vi "Manual_control.vi"() -> ()   [LabVIEW 2015]
uses:
  <vilib>/Instr/_visa.llb/VISA Configure Serial Port (Instr).vi
panel:
  out "Connected to arduino":bool
  out "Heater on":bool
  out "error out":errorcluster
  in  "Tab Control":T1(tab)
  in  "Motor distance (0-999)":string
  in  "Motor speed (NA ATM)":string
  in  "Motor acceleration (00 for constant speed) (NA ATM)":string
  in  "Step type":u16(ring) items=["Sixteenth step", "Eighth step", "Quater step", "Half step", "Full step"]
  in  "Direction":string(combo)
  in  "Motor Trigger":bool
  in  "Apply temp change":bool
  in  "Heater Temperature":string
  in  "Read temp":bool
  out "Recorded temp":string
  in  "Apply changes":bool
  in  "Amplitude set %":dbl(slide) scale=0.0..100.0
  in  "Temprature limit on":bool
  in  "Lower temp limit /°C":dbl
  in  "Upper temp limit /°C":dbl
  in  "Time limit on":bool
  in  "Time limit /s":dbl
  in  "Pluse set %":dbl(slide) scale=0.0..100.0
  in  "Manually turn spray on/off":bool
  in  "Turn off heater":bool
  in  "Stop labview functions.\n To properly disconnect \nfrom arduino use this":bool
  in  "VISA resource name":refnum<visa-resource-name>
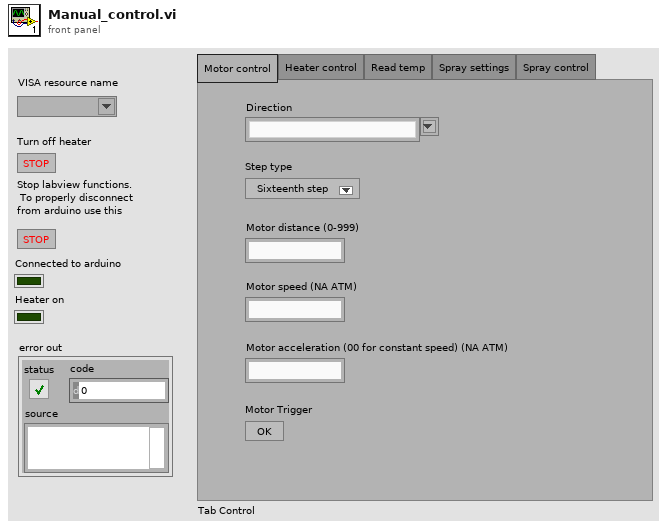
[diagram p1: front panel]
types:
  T1 = enum32{"Motor control", "Heater control", "Read temp", "Spray settings", "Spray control"}
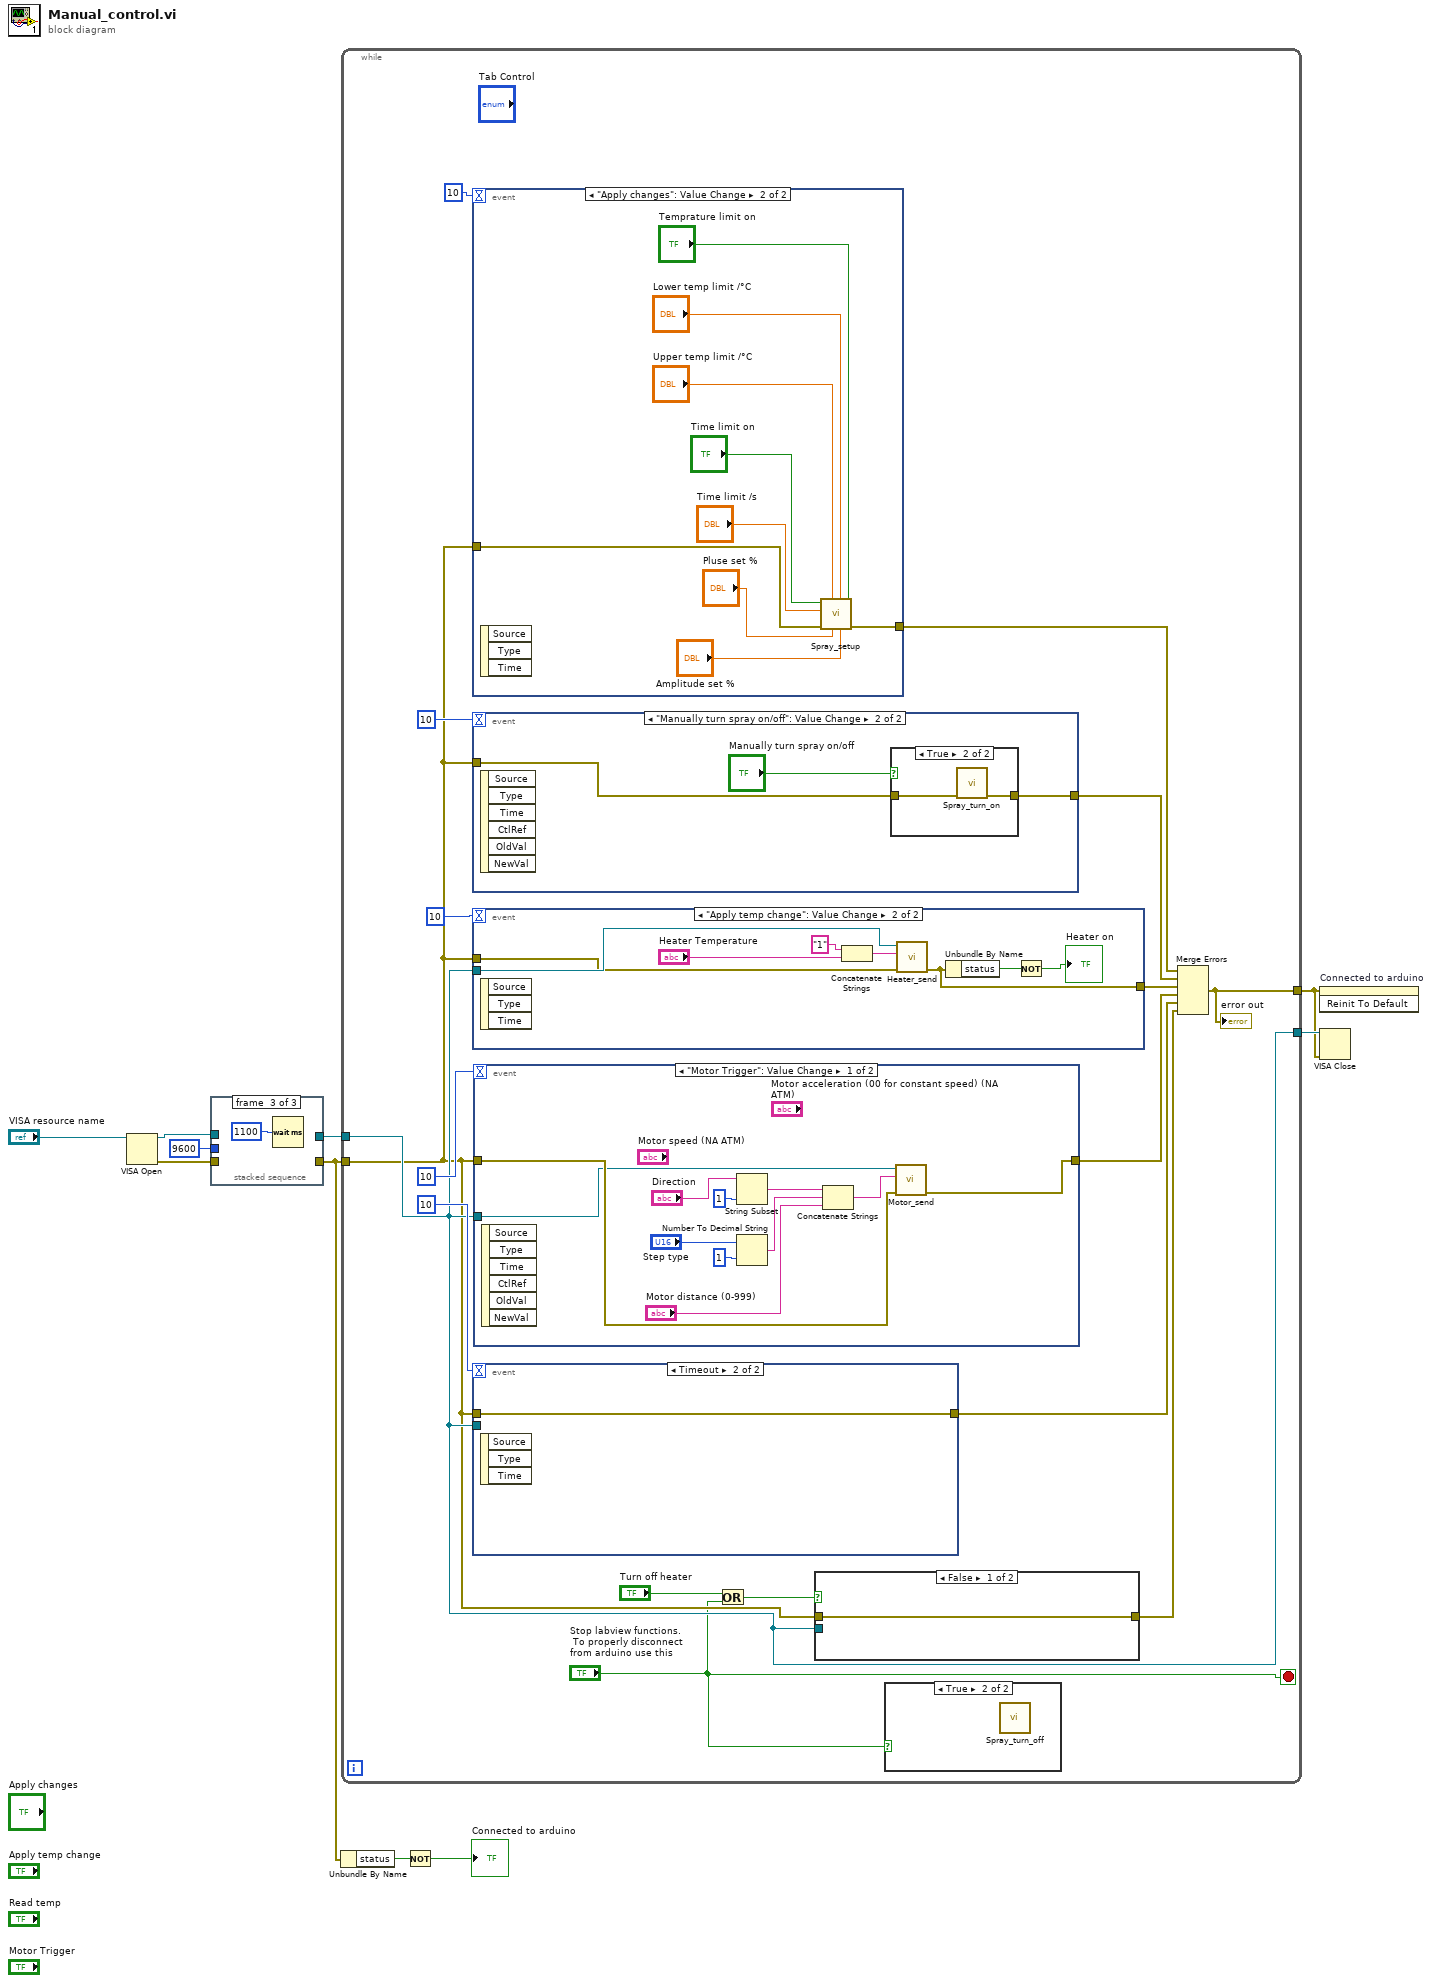
[diagram p0: block diagram]
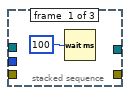
[diagram p2: hidden frame]
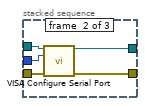
[diagram p3: hidden frame]
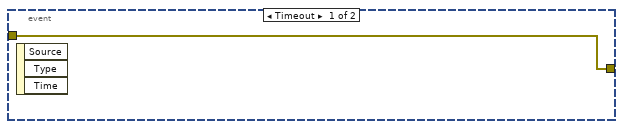
[diagram p5: hidden frame]
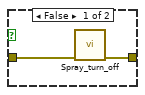
[diagram p6: hidden frame]
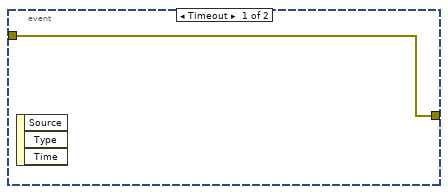
[diagram p7: hidden frame]
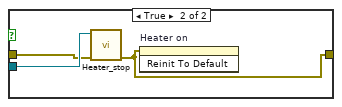
[diagram p8: hidden frame]
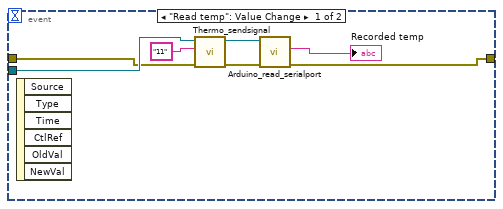
[diagram p9: hidden frame]
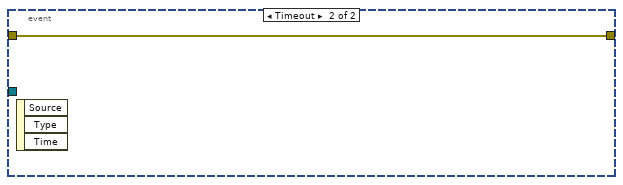
[diagram p10: hidden frame]
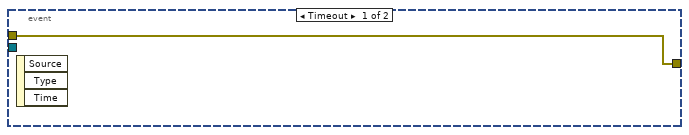
[diagram p11: hidden frame]
diagram:
  n1 = VISA Open(VISA resource name="VISA resource name") -> (VISA resource name=w9:refnum<visa-resource-name>, error out=w8:errorcluster)  [unwired: 4 in]
  n2 = stacked-sequence {
    tunnel: u32 9600 ("baud rate (9600)") -> [_ w16 _]
    tunnel: w9 -> [_ w15 _]
    tunnel: w8 -> [_ w14 _]
    tunnel: [_ w13 _] -> w6
    tunnel: [_ w12 _] -> w4
    frame #0 {
      n3 = Wait (ms)(milliseconds to wait=u32 100) -> ()  [unwired: 1 out]
    }
    frame #1 {
      n4 = call-poly "VISA Configure Serial Port"("VISA resource name"=w15, "baud rate (9600)"=w16, "error in (no error)"=w14) -> ("VISA resource name out"=w13:refnum<visa-resource-name>, "error out"=w12:errorcluster)  [unwired: 11 in]
    }
    frame #2 {
      n5 = Wait (ms)(milliseconds to wait=u32 1100) -> ()  [unwired: 1 out]
    }
  }
  n6 = Unbundle By Name(w4) -> ("status"=w3:bool)
  n7 = while {
    tunnel: w6 -> [w27]
    tunnel: w4 -> [w21]
    tunnel: [w24] -> w1
    tunnel: [w27] -> w5
    stop <- "Stop labview functions.\n To properly disconnect \nfrom arduino use this" stop-if-true
    n8 = event shown="[1] \"Apply changes\": Value Change" {
      selector: _ -> [_ _]
      dyn-events: _ -> [_ _]
      timeout: 10 -> [_ _]
      tunnel: w21 -> [w43 w45]
      tunnel: [w43 w44] -> w19
      event Timeout {
        n9 = event-data() -> ()  [unwired: 1 in, 3 out]
      }
      event "Apply changes": Value Change {
        n10 = event-data() -> ()  [unwired: 1 in, 3 out]
        n11 = call "Spray_setup.vi"("Temp limit on"="Temprature limit on", "Amplitude"="Amplitude set %", "Lower temp limit"="Lower temp limit /°C", "Pulse"="Pluse set %", "Upper temp limit"="Upper temp limit /°C", "error in (no error)"=w45, "Time limit"="Time limit /s", "Time limit on"="Time limit on") -> ("error out"=w44:errorcluster)  [unwired: 3 in]
      }
    }
    n12 = event shown="[1] \"Manually turn spray on/off\": Value Change" {
      selector: _ -> [_ _]
      dyn-events: _ -> [_ _]
      timeout: 10 -> [_ _]
      tunnel: w21 -> [w35 w37]
      tunnel: [w35 w36] -> w20
      event Timeout {
        n13 = event-data() -> ()  [unwired: 1 in, 3 out]
      }
      event "Manually turn spray on/off": Value Change {
        n14 = event-data() -> ()  [unwired: 1 in, 6 out]
        n15 = case shown="True" "Manually turn spray on/off" {
          tunnel: w37 -> [w40 w42]
          tunnel: [w39 w41] -> w36
          frame False {
            n16 = call "Spray_turn_off.vi"("error in (no error)"=w40) -> ("error out"=w39:errorcluster)  [unwired: 10 in]
          }
          frame True {
            n17 = call "Spray_turn_on.vi"("error in (no error)"=w42) -> ("error out"=w41:errorcluster)  [unwired: 10 in]
          }
        }
      }
    }
    n18 = event shown="[1] \"Apply temp change\": Value Change" {
      selector: _ -> [_ _]
      dyn-events: _ -> [_ _]
      timeout: 10 -> [_ _]
      tunnel: [w77 w79] -> w32
      tunnel: w27 -> [_ w82]
      tunnel: w21 -> [w77 w81]
      event Timeout {
        n19 = event-data() -> ()  [unwired: 1 in, 3 out]
      }
      event "Apply temp change": Value Change {
        n20 = event-data() -> ()  [unwired: 1 in, 3 out]
        n21 = Concatenate Strings("1", "Heater Temperature") -> (w83:string)
        n22 = call "Heater_send.vi"("error in (no error)"=w81, "String"=w83, "VISA resource name"=w82) -> ("error out"=w79:errorcluster)  [unwired: 7 in, 1 out]
        n23 = Unbundle By Name(w79) -> ("status"=w80:bool)
        n24 = Not(x=w80) -> (.not. x?=→"Heater on":bool)
      }
    }
    n25 = event shown="[1] Timeout" {
      selector: _ -> [_ _]
      dyn-events: _ -> [_ _]
      timeout: 10 -> [_ _]
      tunnel: w27 -> [w63 _]
      tunnel: w21 -> [w62 w64]
      tunnel: [w58 w64] -> w30
      event "Read temp": Value Change {
        n26 = event-data() -> ()  [unwired: 1 in, 6 out]
        n27 = call "Thermo_sendsignal.vi"("error in (no error)"=w62, "write buffer"="11", "VISA resource name"=w63) -> ("error out"=w59:errorcluster, "VISA resource name out"=w60:refnum<visa-resource-name>)  [unwired: 7 in]
        n28 = call "Arduino_read_serialport.vi"("error in (no error)"=w59, "reference"=w60) -> ("error out"=w58:errorcluster, "String"=→"Recorded temp":string)  [unwired: 6 in, 2 out]
      }
      event Timeout {
        n29 = event-data() -> ()  [unwired: 1 in, 3 out]
      }
    }
    n30 = event shown="[0] \"Motor Trigger\": Value Change" {
      selector: _ -> [_ _]
      dyn-events: _ -> [_ _]
      timeout: 10 -> [_ _]
      tunnel: w21 -> [w68 w76]
      tunnel: w27 -> [w67 _]
      tunnel: [w66 w76] -> w33
      event "Motor Trigger": Value Change {
        n31 = event-data() -> ()  [unwired: 1 in, 6 out]
        n32 = String Subset(string="Direction", length (rest)=1) -> (substring=w65:string)  [unwired: 1 in]
        n33 = Number To Decimal String(number="Step type", width (-)=1) -> (decimal integer string=w71:string)
        n34 = Concatenate Strings(w65, w71, "Motor distance (0-999)") -> (w69:string)
        n35 = call "Motor_send.vi"("error in (no error)"=w68, "String"=w69, "VISA resource name"=w67) -> ("error out"=w66:errorcluster)  [unwired: 7 in, 1 out]
      }
      event Timeout {
        n36 = event-data() -> ()  [unwired: 1 in, 3 out]
      }
    }
    n37 = Or(x="Turn off heater", y="Stop labview functions.\n To properly disconnect \nfrom arduino use this") -> (x .or. y?=w28:bool)
    n38 = case shown="False" w28 {
      tunnel: w27 -> [_ w56]
      tunnel: w21 -> [w53 w55]
      tunnel: [w53 w54] -> w26
      frame False {
      }
      frame True {
        n39 = call "Heater_stop.vi"("error in (no error)"=w55, "VISA resource name"=w56) -> ("error out"=w54:errorcluster)  [unwired: 8 in, 1 out]
        n40 = invoke on="Heater on" class="Bool (strict)" method="Reinit To Default"(error in=w54) -> ()  [unwired: 2 in, 3 out]
      }
    }
    n41 = case shown="True" "Stop labview functions.\n To properly disconnect \nfrom arduino use this" {
      frame False {
      }
      frame True {
        n42 = call "Spray_turn_off.vi"() -> ()  [unwired: 11 in, 1 out]
      }
    }
    n43 = Merge Errors(w19, w20, w32, w33, w30, w26) -> (w24:errorcluster)
    "error out" <- w24
  }
  n44 = Not(x=w3) -> (.not. x?=→"Connected to arduino":bool)
  n45 = invoke on="Connected to arduino" class="Bool (strict)" method="Reinit To Default"(error in=w1) -> ()  [unwired: 2 in, 3 out]
  n46 = VISA Close(VISA resource name=w5, error in (no error)=w1) -> ()  [unwired: 1 out]
